vi "Tell Forward Self.vi"(7 "Actor in":refnum<class "Actor.lvclass">, 9 "Msg DVR":refnum<data-value>) -> (0 "Error out":errorcluster, 5 "Actor out":refnum<class "Actor.lvclass">)   [LabVIEW 2020, in "_Template.lvlib" / "Templates.lvlib" / "TEMPLATE jettl Msg.lvlib"]
uses:
  TEMPLATE jettl Msg.lvlib
  TEMPLATE Msg/TEMPLATE Msg.lvclass
  jettl/jettl/jettl.lvlib
  jettl/jettl/Actor/Actor.lvclass
  jettl/jettl/Msg Contents/Msg Contents.lvclass
  jettl/jettl/Msg/Msg.lvclass
  jettl/jettl/Unified Actor Relation.ctl
  jettl/jettl/Teller.ctl
  jettl/jettl/Msg.ctl
panel:
  # "This front panel should not be manipulated."
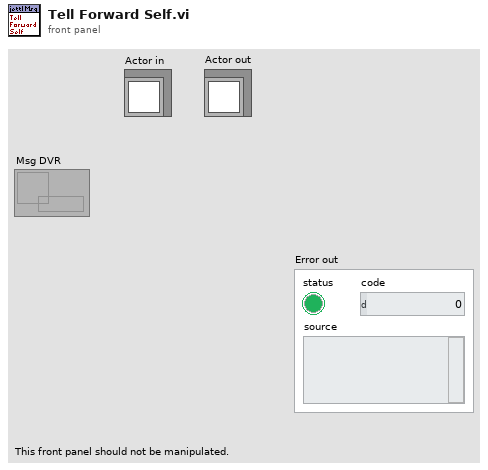
[diagram p1: front panel]
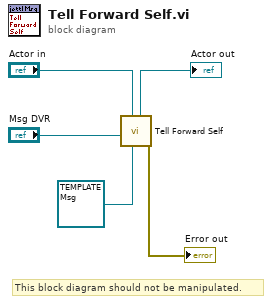
[diagram p0: block diagram]
diagram:
  # "This block diagram should not be manipulated."
  n1 = call "Tell Forward Self.vi"("Msg"=refnum<class "TEMPLATE Msg.lvclass"> refnum ("_Template.lvlib:Templates.lvlib:TEMPLATE jettl Msg.lvlib:TEMPLATE Msg.lvclass"), "Actor in"="Actor in", "Msg DVR"="Msg DVR") -> ("Error out"=→"Error out":errorcluster, "Actor out"=→"Actor out":refnum<class "Actor.lvclass">)  [unwired: 7 in]
